vi "write certain channel value.vi"(0 "Reading channel":T1={"Chan 0"=TRUE, "Chan 1"=TRUE, "Chan 2"=TRUE, "Chan 3"=TRUE}, 1 "FIFO In":refnum<k21>="V FIFO", 5 "Chan 0 value":fxp<+/-,17,5>, 7 "Chan 1 value":fxp<+/-,17,5>, 9 "Chan 2 value":fxp<+/-,17,5>, 11 "Chan 3 value":fxp<+/-,17,5>, 12 "error in (no error)":errorcluster) -> (15 "error out":errorcluster)   [LabVIEW 2023]
uses:
  <vilib>/rvi/DataTransferAndStorage/Container/Common/niFpgaContainerExecOnDevCompGetState.vi
  <vilib>/rvi/Emulation/niFpgaEmulationIsFPGAContextNoSignature.vi
  <vilib>/rvi/Emulation/niFpgaSctlEmulationGetInTimedLoop.vi
  <vilib>/rvi/errors/niFpgaSetErrorForExecOnDevCompSimple.vi
  <vilib>/rvi/eio/common/nirviEmuReportErrorAndStop.vi
  <vilib>/rvi/DataTransferAndStorage/Container/Common/niFpgaContainerGetUniqueNameForEmu.vi
  <vilib>/rvi/FIFO/Fifo_Resource/nirvififoEmulationSetSize.vi
  <vilib>/rvi/FIFO/Fifo_Resource/nirviFifoEmulationQueueMgr.vi
  <instcachedir>/0/nirviFifoEmulationQueueMgr_E5CAEC123FF24DC58D834DCA3CDAA9B5.lvgen/nirviFifoEmulationQueueMgr_E5CAEC123FF24DC58D834DCA3CDAA9B5_001.vi
  <vilib>/rvi/FIFO/Fifo_Resource/nirvififoEmulationDetermineInputValidOut.vi
  <vilib>/rvi/FIFO/Fifo_Resource/nirvififoEmulationCreateLock.vi
  <vilib>/rvi/Emulation/niFpgaProcessEmulError.vi
  <vilib>/rvi/FIFO/Fifo_Resource/nirvififoEmulationObtainLock.vi
  <vilib>/rvi/FIFO/Fifo_Resource/nirvififoEmulationReleaseLock.vi
  <vilib>/rvi/occurrence/nirviWaitOnOccurrenceBase.vi
  <vilib>/rvi/errors/nirviReportUnexpectedCaseInternalError.vi
  <vilib>/rvi/errors/nirviReportUnexpectedCaseInternalError (U32).vi
  <vilib>/Utility/error.llb/Clear Errors.vi
  <vilib>/eio/utilities/niEioResolveVilibRelativePath.vi
  <vilib>/rvi/interface/RandomDataEmulation/niFpgaRandomDataHandleErrors.vi
  <vilib>/rvi/DataTransferAndStorage/Container/XNode/niFpgaContainer.xnode
  <vilib>/rvi/FIFO/Fifo_Resource/niFpgaFifoEmulationRefIn.vi
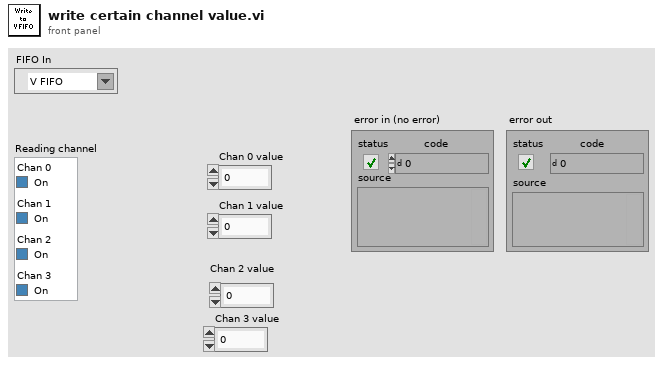
[diagram p1: front panel]
types:
  T1 = cluster{"Chan 0":bool, "Chan 1":bool, "Chan 2":bool, "Chan 3":bool}
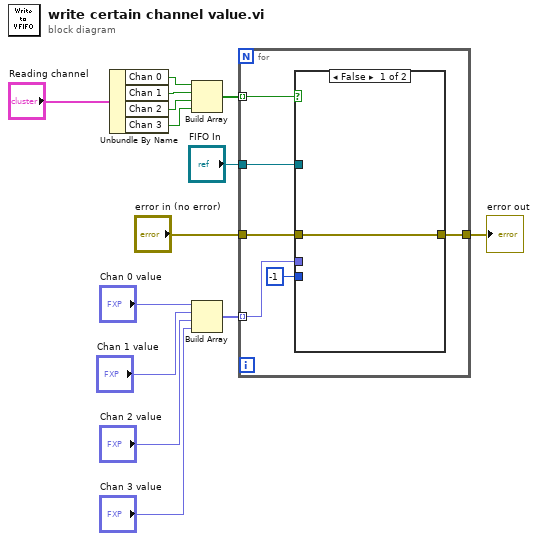
[diagram p0: block diagram]
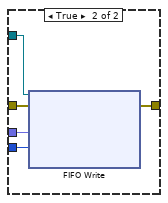
[diagram p2: hidden frame]
diagram:
  n1 = Unbundle By Name("Reading channel") -> ("Chan 0"=w10:bool, "Chan 1"=w9:bool, "Chan 2"=w8:bool, "Chan 3"=w7:bool)
  n2 = Build Array(w10, w9, w8, w7) -> (w6:bool[])
  n3 = Build Array("Chan 0 value", "Chan 1 value", "Chan 2 value", "Chan 3 value") -> (w1:fxp<+/-,17,5>[])
  n4 = for {
    tunnel: "error in (no error)" -> [w19]
    tunnel: "FIFO In" -> [w18]
    tunnel: [w17] -> w11
    tunnel: w6 -> [w16] mode=indexing
    tunnel: w1 -> [w15] mode=indexing
    n5 = case shown="False" w16 {
      tunnel: -1 ("Timeout") -> [_ w26]
      tunnel: w19 -> [w21 w25]
      tunnel: w18 -> [_ w24]
      tunnel: [w21 w23] -> w17
      tunnel: w15 -> [_ w22]
      frame False {
      }
      frame True {
        n6 = xnode ("FIFO Write")("Element"=w22, "Timeout"=w26, "error in (no error)"=w25, "FIFO In"=w24) -> ("error out"=w23:errorcluster)  [unwired: 2 out]
      }
    }
  }
  "error out" <- w11
